vi "Get Item Info.vi"(8 "error in (no error)":errorcluster, 11 "Object":T1) -> (0 "error out":errorcluster, 1 "Item Refnum":refnum<vi>, 2 "Target":refnum<vi>, 3 "Object":T1, 4 "Project Path":path)   [LabVIEW 2020, in "Message Maker Provider.lvlib"]
uses:
  Message Maker Provider.lvlib
  <resource>/Framework/Providers/API/ItemRef.ctl
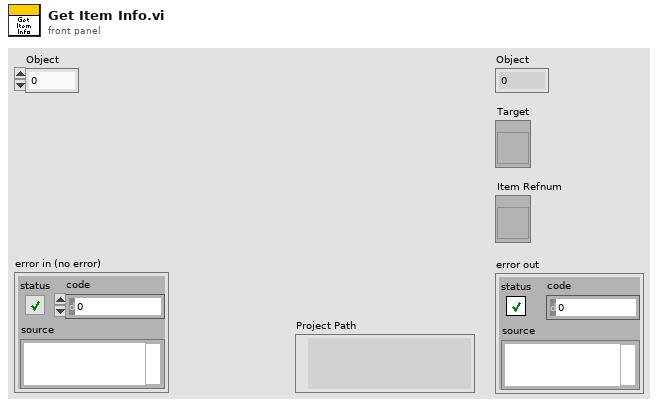
[diagram p1: front panel]
types:
  T1 = typedef "ItemRef.ctl" = u64
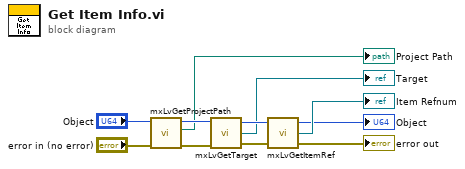
[diagram p0: block diagram]
diagram:
  n1 = call <resource>:"mxLvGetProjectPath.vi"("error in"="error in (no error)", "Item"="Object") -> ("error out"=w7:errorcluster, "Project Path"=→"Project Path":path, "Item"=w9:T1)  [unwired: 7 in]
  n2 = call <resource>:"mxLvGetTarget.vi"("Item"=w9, "error in"=w7) -> ("Item"=w6:T1, "Target"=→"Target":refnum<vi>, "error out"=w8:errorcluster)
  n3 = call <resource>:"mxLvGetItemRef.vi"("Item"=w6, "error in"=w8) -> ("Item"=→"Object":T1, "Item Refnum"=→"Item Refnum":refnum<vi>, "error out"=→"error out":errorcluster)
